vi "init control_path.vi"(8 "error in (no error)":errorcluster, 10 "Path Refnum":refnum<vi>) -> (0 "error out":errorcluster, 3 "Control out":refnum<class "Control.lvclass">)   [LabVIEW 2010, in "Control.lvclass"]
uses:
  Control.lvclass
  Path Control/Path Control.lvclass
  Control.lvclass/Control.ctl
panel:
  in  "Control in":refnum<class "Control.lvclass">
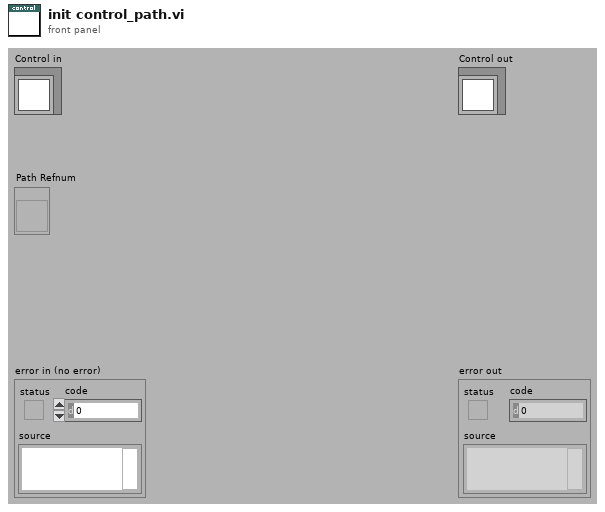
[diagram p1: front panel]
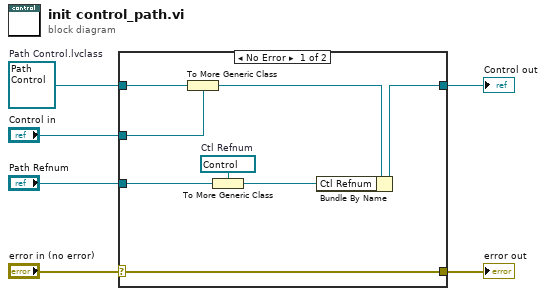
[diagram p0: block diagram]
diagram:
  w1 = refnum<class "Path Control.lvclass"> refnum  # Path Control.lvclass
  n1 = case shown="No Error" "error in (no error)" {
    selector: "error in (no error)" -> [w14 w16]
    tunnel: [w14 w16] -> w5
    tunnel: [w13 w15] -> w3
    tunnel: "Control in" -> [w8 w15]
    tunnel: "Path Refnum" -> [w12 _]
    tunnel: w1 -> [w9 _]
    frame No Error {
      w10 = refnum<vi> refnum  # Ctl Refnum
      n2 = To More Generic Class(target class=w8, reference=w9) -> (generic class reference=w7:refnum<class "Control.lvclass">)
      n3 = To More Generic Class(target class=w10, reference=w12) -> (generic class reference=w11:refnum<vi>)
      n4 = Bundle By Name(cluster=w7, "Ctl Refnum"=w11) -> (w13:refnum<class "Control.lvclass">)
    }
    frame Error {
    }
  }
  "error out" <- w5
  "Control out" <- w3
